vi "Acquisition_Thermal.vi"() -> ()   [LabVIEW 2010]
uses:
  <vilib>/Utility/error.llb/DialogType.ctl
  Types/TYPE Filter Outputs.ctl
  <vilib>/DAQmx/read.llb/DAQmx Read (Analog 1D Wfm NChan NSamp).vi
  <vilib>/daqmx/miscellaneous.llb/DAQmx Fill In Error Info.vi
  <vilib>/Utility/file.llb/Write To Spreadsheet File (DBL).vi
panel:
  in  "Modeling:":u16(ring) items=["Initial", "Repeat"]
  in  "Preamp Gain":u16(ring)=10 items=["10X"=10, "100X"=100]
  in  "Q Interval":i32=600
  in  "Stop":bool
  in  "Feature Save To Path":path=path "C:/Users/local_admin/Desktop/Sleep Modulation - 08012016/Spiny9_0803.csv"
  out "Target Temp":dbl
  out "Temp":dbl
  out "Q":dbl
  out "T < Target":bool
  in  "EEG Coefficients File":path=path "C:/Users/local_admin/Desktop/Sleep Modulation - 08012016/EEG_Coefs.csv"
  in  "Model Information (Mu, Sigma, Priors, Transition Matrix):":path=path "C:/Users/local_admin/Desktop/Sleep Modulation - 08012016/Model_Spiny9_0801_2.csv"
  out "Sleep Stage":i32
  out "EEG":waveform(dbl)(graph)
  out "EMG":waveform(dbl)(graph)
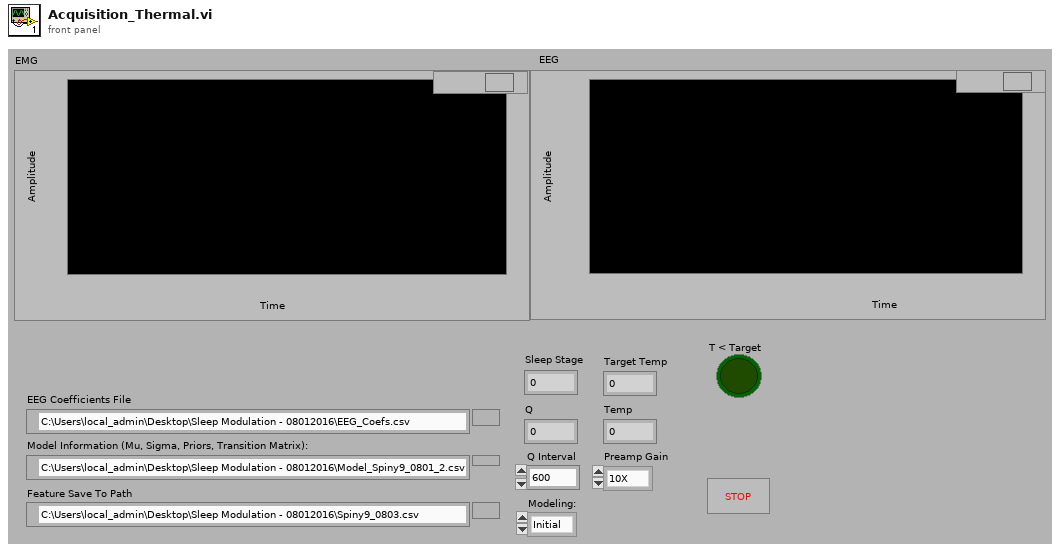
[diagram p1: front panel]
types:
  T1 = typedef "DialogType.ctl" = u16
  T2 = typedef "TYPE Filter Outputs.ctl" = cluster{"Delta:Theta":dbl, "Hi:Lo":dbl, "EMG":dbl, "Delta Low":dbl, "Theta":dbl, "Alpha":dbl, "Beta":dbl, "Gamma":dbl, "Total EEG":dbl, "Detection":dbl, "Stimulate":dbl, "TimeStamp":dbl, "Class Labels":dbl, "Delta High":dbl}
  T3 = typedef "TYPE EEG Components.ctl" = cluster{"Total":dbl, "Alpha":dbl, "Beta":dbl, "Gamma":dbl, "Delta":dbl, "Delta Low":dbl, "Delta High":dbl, "Theta":dbl}
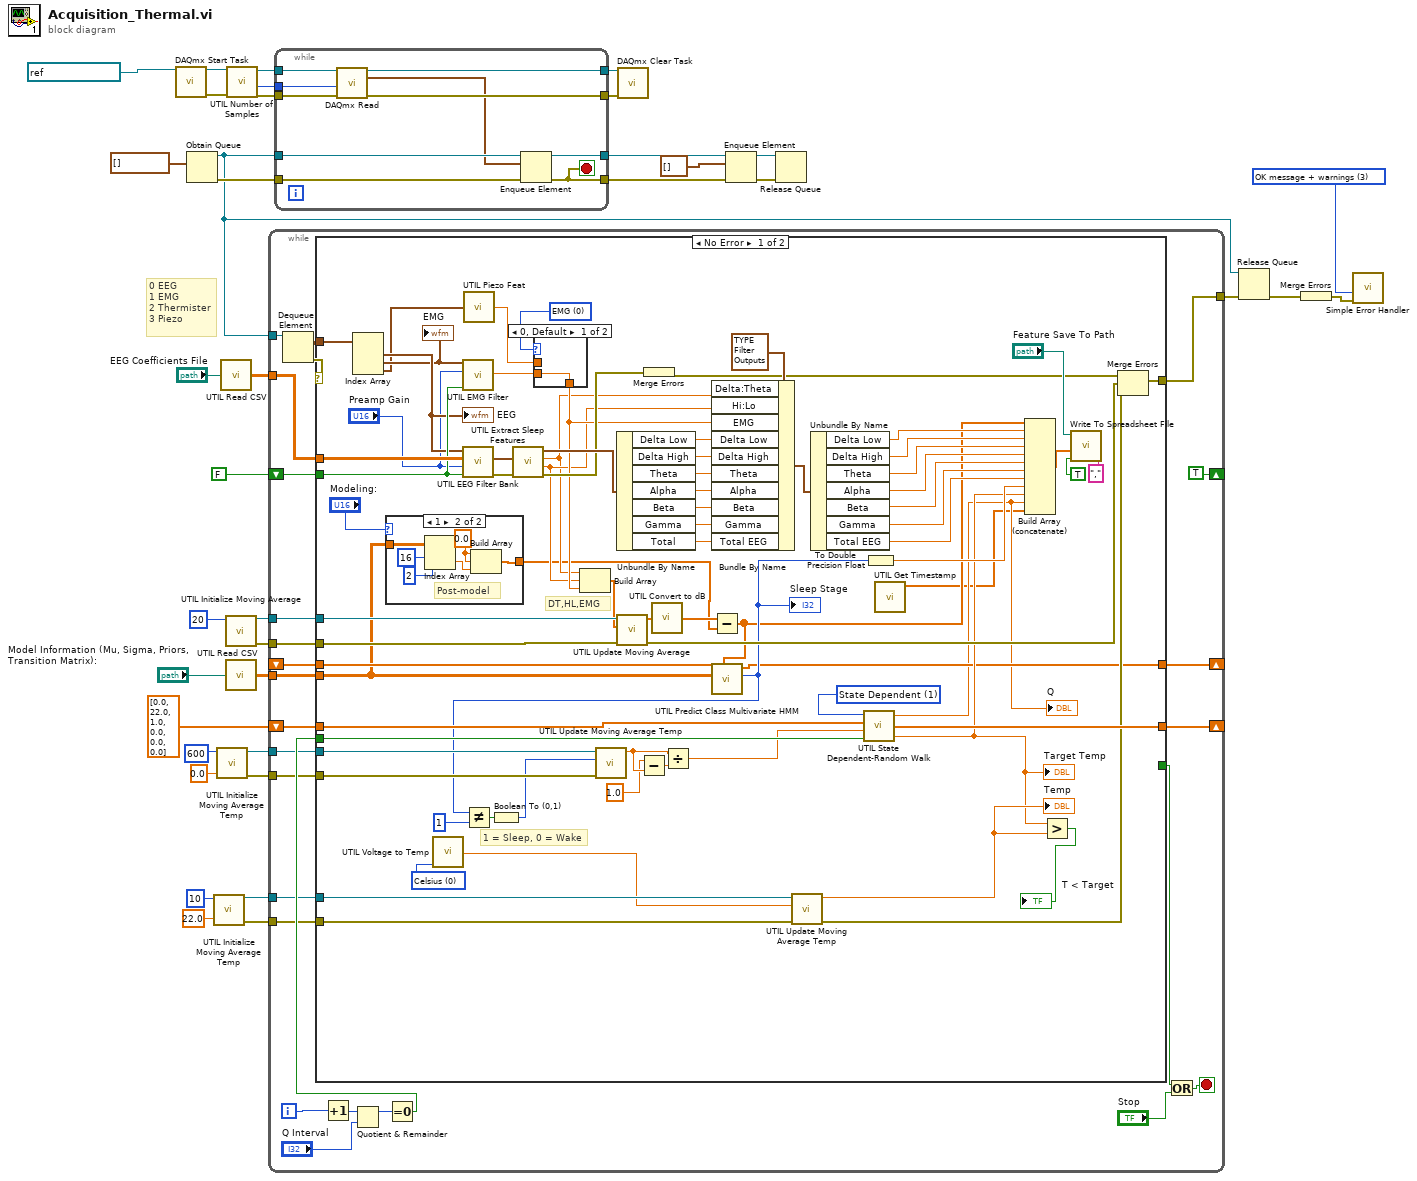
[diagram p0: block diagram]
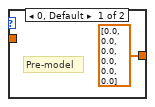
[diagram p2: hidden frame]
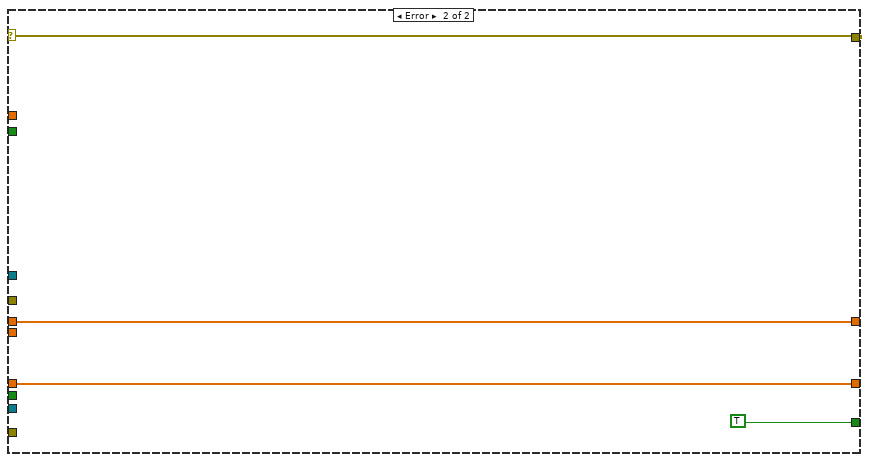
[diagram p4: hidden frame]
diagram:
  w30 = T1 3 items=["no dialog", "OK message", "continue or stop message", "OK message + warnings", "continue/stop + warnings"] ("type of dialog (OK msg:1)")
  # "0 EEG\n1 EMG\n2 Thermister\n3 Piezo"
  n1 = call <vilib>:"DAQmx Start Task.vi"("task/channels in"=refnum<k21> "SEGWAY_RT") -> ("task out"=w21:refnum<k21>, "error out"=w20:errorcluster)  [unwired: 13 in]
  n2 = Obtain Queue(element data type=waveform(dbl)[] [] ("Measurement 2")) -> (queue out=w28:refnum<queue>, error out=w36:errorcluster)  [unwired: 4 in, 1 out]
  n3 = call "UTIL Initialize Moving Average Temp.vi"("element"=22.0, "Window Width"=10) -> ("Error Out"=w8:errorcluster, "queue out"=w9:refnum<queue>)  [unwired: 8 in]
  n4 = call "UTIL Initialize Moving Average Temp.vi"("element"=0.0, "Window Width"=600) -> ("Error Out"=w5:errorcluster, "queue out"=w6:refnum<queue>)  [unwired: 8 in]
  n5 = call "UTIL Read CSV.vi"("CSV Path"="EEG Coefficients File") -> ("Data From File"=w2:dbl[][])
  n6 = call "UTIL Initialize Moving Average.vi"("Window Width"=20) -> ("Error Out"=w13:errorcluster, "queue out"=w11:refnum<queue>)  [unwired: 9 in]
  n7 = call "UTIL Read CSV.vi"("CSV Path"="Model Information (Mu, Sigma, Priors, Transition Matrix):") -> ("Data From File"=w25:dbl[][])
  n8 = call "UTIL Number of Samples.vi"("Error In"=w20, "Task In"=w21) -> ("Error Out"=w16:errorcluster, "Samples/Chan"=w17:i32, "Task Out"=w18:refnum<k21>)  [unwired: 7 in]
  n9 = while {
    tunnel: w28 -> [w61]
    shift-right: [TRUE] -> _
    shift-left: FALSE -> [w59]
    tunnel: [w53] -> w27
    tunnel: w13 -> [w56]
    tunnel: w25 -> [w55]
    tunnel: w2 -> [w54]
    shift-right: [w51] -> _
    shift-left: dbl[] [0.0, 22.0, 1.0, 0.0, 0.0, 0.0] ("Parameters Out") -> [w50]
    tunnel: w11 -> [w46]
    tunnel: w9 -> [w45]
    tunnel: w8 -> [w44]
    tunnel: w6 -> [w41]
    tunnel: w5 -> [w40]
    shift-right: [w39] -> _
    shift-left: _ -> [w38]
    i -> [w48]
    stop <- w58 stop-if-true
    n10 = Dequeue Element(queue=w61) -> (element=w62:waveform(dbl)[], error out=w63:errorcluster)  [unwired: 2 in, 2 out]
    n11 = Increment(x=w48) -> (x+1=w49:i32)
    n12 = Quotient & Remainder(x=w49, y="Q Interval") -> (x-y*floor(x/y)=w52:i32)  [unwired: 1 out]
    n13 = Equal To 0?(x=w52) -> (x = 0?=w47:bool)
    n14 = case shown="No Error" w63 {
      selector: w63 -> [_ w151]
      tunnel: w62 -> [w72 _]
      tunnel: w59 -> [w108 _]
      tunnel: [_ TRUE] -> w57
      tunnel: [w114 w151] -> w53
      tunnel: w56 -> [w105 _]
      tunnel: w55 -> [w71 _]
      tunnel: w54 -> [w110 _]
      tunnel: w47 -> [w113 _]
      tunnel: [w112 w150] -> w51
      tunnel: w50 -> [w97 w150]
      tunnel: w46 -> [w103 _]
      tunnel: w45 -> [w102 _]
      tunnel: w44 -> [w99 _]
      tunnel: w41 -> [w96 _]
      tunnel: w40 -> [w95 _]
      tunnel: [w83 w149] -> w39
      tunnel: w38 -> [w82 w149]
      frame No Error {
        w79 = u16 0 items=["EMG", "Piezo", ""] ("Temperature Units (C)")
        w86 = u16 1 items=["Random Walk", "State Dependent"] ("Temperature Units (C)")
        w111 = u16 0 items=["Celsius", "Fahrenheit", "Kelvin", "Rankine"] ("Temperature Units (C)")
        # "1 = Sleep, 0 = Wake"
        # "DT,HL,EMG"
        n15 = Index Array(array=w72) -> (element #1=w107:waveform(dbl), element #2=w106:waveform(dbl), element #3=w64:waveform(dbl))  [unwired: 3 in]
        "EMG" <- w106
        "EEG" <- w107
        n16 = case shown="1" "Modeling:" {
          tunnel: w71 -> [_ w146]
          tunnel: [dbl[] [0.0, 0.0, 0.0, 0.0, 0.0, 0.0] ("Parameters Out") w145] -> w69
          frame 0, Default {
            # "Pre-model"
          }
          frame 1 {
            w141 = 0.0 ("element")
            # "Post-model"
            n17 = Index Array(array=w146, index (row)=16, index (col)=2 ("disabled index (col)")) -> (element=w142:dbl)
            n18 = Build Array(w141, w141, w142) -> (w145:dbl[])
          }
        }
        n19 = call "UTIL Voltage to Temp.vi"("Temperature Units (C)"=w111) -> ("Temp"=w101:dbl)  [unwired: 10 in]
        n20 = call "UTIL EMG Filter.vi"("init/cont (init:F)"=w108, "Preamp Gain"="Preamp Gain", "EMG In"=w106) -> ("EMG Power"=w81:dbl)  [unwired: 7 in, 1 out]
        n21 = call "UTIL EEG Filter Bank.vi"("init/cont (init:F)"=w108, "Amplifier Gain"="Preamp Gain", "Filter Coefficients from File"=w110, "EEG In"=w107) -> ("Error Out"=w139:errorcluster, "EEG Components"=w109:T3)  [unwired: 5 in, 1 out]
        n22 = call "UTIL Piezo Feat.vi"("Piezo In"=w64) -> ("Piezo Power"=w80:dbl)  [unwired: 4 in]
        n23 = call "UTIL Extract Sleep Features.vi"("Error In"=w139, "Components In"=w109) -> ("Error Out"=w125:errorcluster, "Hi:Lo"=w76:dbl, "Delta:Theta"=w75:dbl, "Components Out"=w137:T3)  [unwired: 6 in]
        n24 = case shown="0, Default" w79 {
          tunnel: w81 -> [w147 _]
          tunnel: w80 -> [_ w148]
          tunnel: [w147 w148] -> w77
          frame 0, Default {
          }
          frame 1 {
          }
        }
        n25 = Build Array(w75, w76, w77) -> (w74:dbl[])
        n26 = Unbundle By Name(w137) -> ("Delta Low"=w124:dbl, "Delta High"=w123:dbl, "Theta"=w122:dbl, "Alpha"=w121:dbl, "Beta"=w120:dbl, "Gamma"=w119:dbl, "Total"=w118:dbl)
        n27 = call "UTIL Update Moving Average.vi"("Error In"=w105, "Data In"=w74, "Average Queue"=w103) -> ("Error Out"=w104:errorcluster, "Average"=w73:dbl[])  [unwired: 7 in]
        n28 = Merge Errors(w125) -> (w115:errorcluster)
        n29 = call "UTIL Convert to dB.vi"("Features In"=w73) -> ("Features (dB)"=w70:dbl[])
        n30 = Bundle By Name(cluster=T2 {"Delta:Theta"=0.0, "Hi:Lo"=0.0, "EMG"=0.0, "Delta Low"=0.0, "Theta"=0.0, "Alpha"=0.0, "Beta"=0.0, "Gamma"=0.0, "Total EEG"=0.0, "Detection"=0.0, "Stimulate"=0.0, "TimeStamp"=0.0, "Class Labels"=0.0, "Delta High"=0.0} ("Filter Outputs"), "Delta:Theta"=w75, "Hi:Lo"=w76, "EMG"=w77, "Delta Low"=w124, "Delta High"=w123, "Theta"=w122, "Alpha"=w121, "Beta"=w120, "Gamma"=w119, "Total EEG"=w118) -> (w136:T2)
        n31 = Subtract(x=w70, y=w69) -> (x-y=w67:dbl[])
        n32 = call "UTIL Predict Class Multivariate HMM.vi"("Data Point"=w67, "Model Information"=w71, "d(t-1) In"=w82) -> ("Sleep Stage"=w84:i32, "d(t-1) Out"=w83:dbl[])  [unwired: 5 in]
        "Sleep Stage" <- w84
        n33 = Not Equal?(x=w84, y=1) -> (x != y?=w93:bool)
        n34 = Boolean To (0,1)(Boolean=w93) -> (0, 1=w92:i16)
        n35 = call "UTIL Update Moving Average Temp.vi"("Error In"=w95, "Data Point"=w92, "Average Queue"=w96) -> ("Moving Average"=w90:dbl)  [unwired: 7 in, 1 out]
        n36 = Subtract(x=1.0, y=w90) -> (x-y=w91:dbl)
        n37 = Divide(x=w90, y=w91) -> (x/y=w88:dbl)
        n38 = call "UTIL Update Moving Average Temp.vi"("Error In"=w99, "Data Point"=w101, "Average Queue"=w102) -> ("Error Out"=w98:errorcluster, "Moving Average"=w100:dbl)  [unwired: 7 in]
        "Temp" <- w100
        n39 = Unbundle By Name(w136) -> ("Delta Low"=w135:dbl, "Delta High"=w127:dbl, "Theta"=w128:dbl, "Alpha"=w129:dbl, "Beta"=w130:dbl, "Gamma"=w134:dbl, "Total EEG"=w117:dbl)
        n40 = call "UTIL State Dependent-Random Walk.vi"("Boolean"=w113, "Numeric"=w88, "Parameters Out"=w97, "Temperature Units (C)"=w86) -> ("Target Temp"=w85:dbl, "Parameters Out"=w112:dbl[], "Q"=w66:dbl)
        "Q" <- w66
        "Target Temp" <- w85
        n41 = To Double Precision Float(number=w84) -> (double precision float=w116:dbl)
        n42 = call "UTIL Get Timestamp.vi"() -> ("appended array"=w65:dbl[])  [unwired: 7 in, 1 out]
        n43 = Build Array (concatenate)(w67, w135, w127, w128, w129, w130, w134, w117, w116, w85, w66, w65) -> (w126:dbl[])
        n44 = Greater?(x=w85, y=w100) -> (0:→"T < Target":bool)
        n45 = call-poly <vilib>:"Write To Spreadsheet File.vi"("delimiter (\\t)"="," ("delimiter (\\t)"), "append to file? (new file:F)"=TRUE, "1D data"=w126, "file path (dialog if empty)"="Feature Save To Path") -> ()  [unwired: 4 in, 1 out]
        n46 = Merge Errors(w115, w104, w98) -> (w114:errorcluster)
      }
      frame Error {
      }
    }
    n47 = Or(x=w57, y="Stop") -> (x .or. y?=w58:bool)
  }
  n48 = while {
    tunnel: [w162] -> w15
    tunnel: w28 -> [w161]
    tunnel: w36 -> [w160]
    tunnel: [w159] -> w34
    tunnel: [w158] -> w33
    tunnel: w18 -> [w157]
    tunnel: w17 -> [w156]
    tunnel: w16 -> [w155]
    tunnel: [w154] -> w14
    stop <- w158 stop-if-true
    n49 = call-poly <vilib>:"DAQmx Read.vi"("task/channels in"=w157, "number of samples per channel"=w156, "error in"=w155) -> ("task out"=w162:refnum<k21>, "data"=w153:waveform(dbl)[], "error out"=w154:errorcluster)  [unwired: 10 in]
    n50 = Enqueue Element(queue=w161, element=w153, error in (no error)=w160) -> (queue out=w159:refnum<queue>, error out=w158:errorcluster)  [unwired: 1 in, 1 out]
  }
  n51 = call <vilib>:"DAQmx Clear Task.vi"("task in"=w15, "error in"=w14) -> ()  [unwired: 13 in, 1 out]
  n52 = Enqueue Element(queue=w34, element=waveform(dbl)[] [] ("Measurement 2"), error in (no error)=w33) -> (queue out=w31:refnum<queue>, error out=w29:errorcluster)  [unwired: 1 in, 1 out]
  n53 = Release Queue(queue=w31, error in (no error)=w29) -> ()  [unwired: 1 in, 3 out]
  n54 = Release Queue(queue=w28, error in (no error)=w27) -> (error out=w22:errorcluster)  [unwired: 1 in, 2 out]
  n55 = Merge Errors(w22) -> (w23:errorcluster)
  n56 = call <vilib>:"Simple Error Handler.vi"("type of dialog (OK msg:1)"=w30, "error in (no error)"=w23) -> ()  [unwired: 3 in, 5 out]
